vi "485测试事件结构.vi"() -> ()   [LabVIEW 2018]
doc: "本范例可设置指定端口的RS-485收发器控制模式，并实现串口读取、串口写入或串口读写操作。如果选择全部，VI将写入数据并读取数据，然后关闭开放给端口的VISA会话句柄。该VI将等待直到端口接收到指定的字节数或者接收到终止符。本范例仅适用于NI RS-485接口。\n\n范例演示了使用NI RS-485产品时可用的收发器控制模式。通过RS-485连接一个或多个设备时，用户可能需要减少连线数量。或者用户需要匹配部分设备提供的连线配置。根据连接串行设备所需的连线方式可确定NI RS-485收发器控制模式。\n\n与双线设备进行通信时，National Instruments建议使用双线自动控制模式。该模式可处理硬件中两线连接的发送器/接收器启用模式，因此可减少应用程序中执行该操作的软件开销。"
uses:
  <vilib>/Instr/_visa.llb/VISA Configure Serial Port (Instr).vi
panel:
  in  "时":dbl
  in  "分":dbl
  out "日期":string
  out "时间":string
  out "字符串":string
  in  "秒":dbl
  in  "停止 3":bool
  out "Serial Settings:Number of Bytes at Serial Port 5":u32
  in  "关闭全部继电器":bool=TRUE
  out "Serial Settings:Number of Bytes at Serial Port 4":u32
  in  "打开全部继电器":bool=TRUE
  out "Serial Settings:Number of Bytes at Serial Port 3":u32
  out "数字 2":u32
  out "数字":u32
  in  "停止":bool
  out "读取缓冲区":string
  in  "串口设置":T1={"baud rate"=9600, "data bits"=8, "parity"=enum."None", "stop bits"=10, "flow control"=0} {"flow control" items=["无"=0, "XON/XOFF"=1, "RTS/CTS"=2, "DTR/DSR"=4]; "stop bits" items=["1.0"=10, "1.5"=15, "2.0"=20]; "data bits" min=5 max=8 step=1; "baud rate" items=["75"=75, "110"=110, "134"=134, "150"=150, "300"=300, "600"=600, "1200"=1200, "1800"=1800, "2400"=2400, "4800"=4800, "7200"=7200, "9600"=9600, "14400"=14400, "19200"=19200, "28800"=28800, "38400"=38400, "56000"=56000, "57600"=57600, "115200"=115200, "128000"=128000, "230400"=230400]}
  in  "VISA RS 485资源":refnum<visa-resource-name>="COM1"
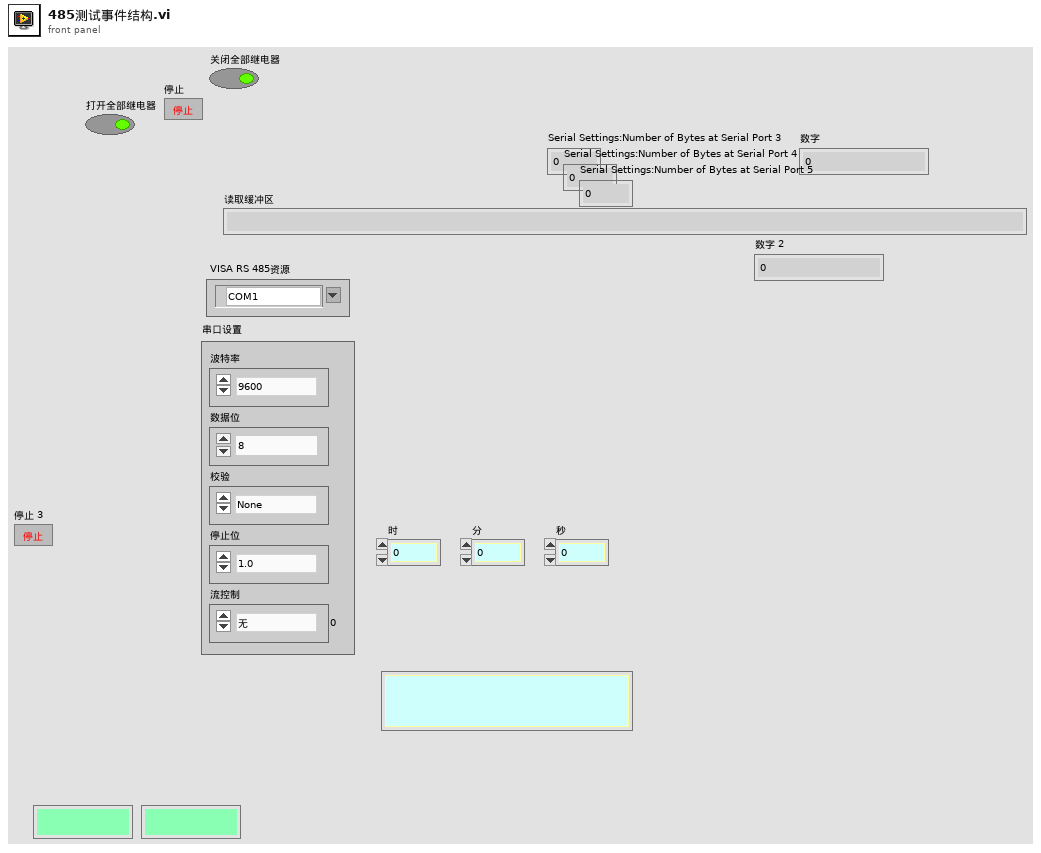
[diagram p1: front panel]
types:
  T1 = typedef "Serial - Settings.ctl" = cluster{"baud rate":u32, "data bits":u16, "parity":enum16{"None", "Odd", "Even", "Mark", "Space"}, "stop bits":u16, "flow control":u16}
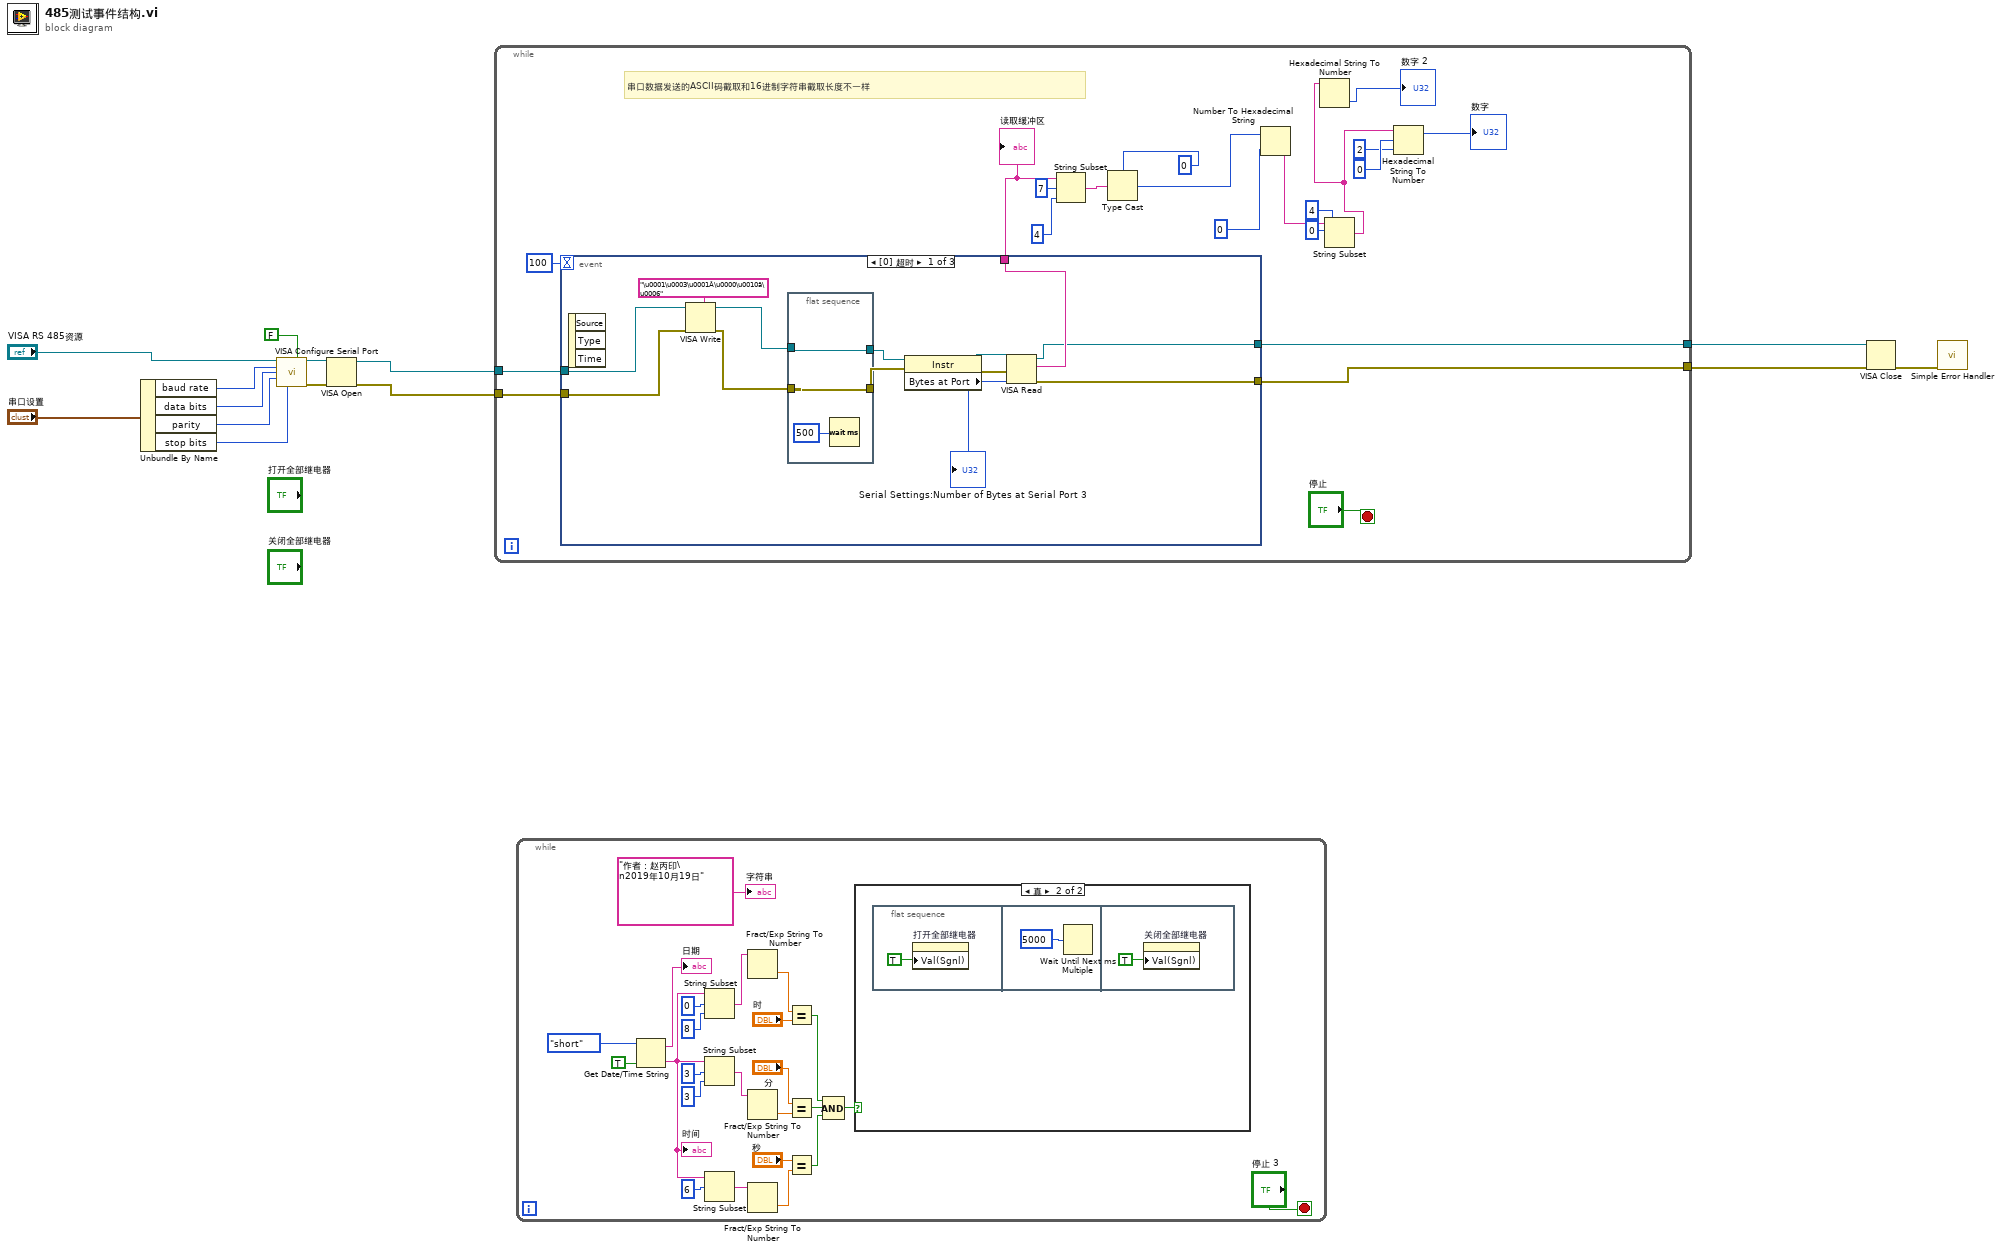
[diagram p0: block diagram]
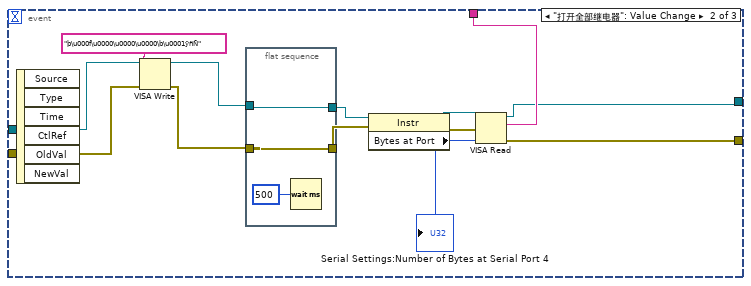
[diagram p3: hidden frame]
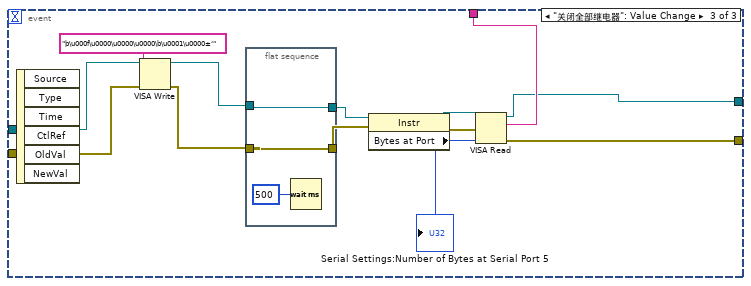
[diagram p4: hidden frame]
diagram:
  n1 = Unbundle By Name("串口设置") -> ("baud rate"=w12:u32, "data bits"=w11:u16, "parity"=w10:enum16{"None", "Odd", "Even", "Mark", "Space"}, "stop bits"=w9:u16)
  n2 = call-poly "VISA Configure Serial Port"("VISA resource name"="VISA RS 485资源", "Enable Termination\nChar (T)"=FALSE ("Enable Termination\nChar (T)"), "baud rate (9600)"=w12, "data bits (8)"=w11, "parity (0:none)"=w10, "stop bits (10: 1 bit)"=w9) -> ("VISA resource name out"=w3:refnum<visa-resource-name>, "error out"=w4:errorcluster)  [unwired: 3 in, 5 out]
  n3 = VISA Open(error in (no error)=w4, VISA resource name=w3) -> (VISA resource name=w1:refnum<visa-resource-name>, error out=w2:errorcluster)  [unwired: 3 in]
  n4 = while {
    tunnel: [w23] -> w6
    tunnel: [w22] -> w5
    tunnel: w2 -> [w18]
    tunnel: w1 -> [w17]
    stop <- "停止" stop-if-true
    # "串口数据发送的ASCII码截取和16进制字符串截取长度不一样"
    n5 = event shown="[0] 超时" {
      selector: _ -> [_ _ _]
      dyn-events: _ -> [_ _ _]
      timeout: 100 -> [_ _ _]
      tunnel: [w48 w64 w80] -> w34
      tunnel: [w47 w52 w68] -> w23
      tunnel: [w46 w53 w69] -> w22
      tunnel: w18 -> [w45 w63 w79]
      tunnel: w17 -> [w44 w62 w78]
      event Timeout {
        n6 = event-data() -> ()  [unwired: 1 in, 3 out]
        n7 = VISA Write(VISA resource name=w44, write buffer="\u0001\u0003\u0001Â\u0000\u0010ä\u0006" ("写入字符串 3"), error in (no error)=w45) -> (VISA resource name out=w39:refnum<visa-resource-name>, error out=w37:errorcluster)  [unwired: 1 out]
        n8 = flat-sequence {
          tunnel: w39 -> [w51]
          tunnel: [w51] -> w38
          tunnel: w37 -> [w50]
          tunnel: [w50] -> w36
          frame #0 {
            n9 = Wait (ms)(milliseconds to wait=u32 500 ("等待时间（毫秒）")) -> ()  [unwired: 1 out]
          }
        }
        n10 = property class="Instr"(reference=w38, error in=w36) -> (reference out=w41:refnum<visa-resource-name>, error out=w40:errorcluster, "Bytes at Port"=w42:u32)
        "Serial Settings:Number of Bytes at Serial Port 3" <- w42
        n11 = VISA Read(VISA resource name=w41, byte count=w42, error in (no error)=w40) -> (VISA resource name out=w46:refnum<visa-resource-name>, read buffer=w48:string, error out=w47:errorcluster)  [unwired: 1 out]
      }
      event "打开全部继电器": Value Change {
        n12 = event-data() -> ()  [unwired: 1 in, 6 out]
        n13 = VISA Write(VISA resource name=w62, write buffer="þ\u000f\u0000\u0000\u0000\b\u0001ÿñÑ" ("写入字符串 3"), error in (no error)=w63) -> (VISA resource name out=w57:refnum<visa-resource-name>, error out=w55:errorcluster)  [unwired: 1 out]
        n14 = flat-sequence {
          tunnel: w57 -> [w67]
          tunnel: [w67] -> w56
          tunnel: w55 -> [w66]
          tunnel: [w66] -> w54
          frame #0 {
            n15 = Wait (ms)(milliseconds to wait=u32 500 ("等待时间（毫秒）")) -> ()  [unwired: 1 out]
          }
        }
        n16 = property class="Instr"(reference=w56, error in=w54) -> (reference out=w59:refnum<visa-resource-name>, error out=w58:errorcluster, "Bytes at Port"=w60:u32)
        "Serial Settings:Number of Bytes at Serial Port 4" <- w60
        n17 = VISA Read(VISA resource name=w59, byte count=w60, error in (no error)=w58) -> (VISA resource name out=w53:refnum<visa-resource-name>, read buffer=w64:string, error out=w52:errorcluster)  [unwired: 1 out]
      }
      event "关闭全部继电器": Value Change {
        n18 = event-data() -> ()  [unwired: 1 in, 6 out]
        n19 = VISA Write(VISA resource name=w78, write buffer="þ\u000f\u0000\u0000\u0000\b\u0001\u0000±‘" ("写入字符串 3"), error in (no error)=w79) -> (VISA resource name out=w73:refnum<visa-resource-name>, error out=w71:errorcluster)  [unwired: 1 out]
        n20 = flat-sequence {
          tunnel: w73 -> [w83]
          tunnel: [w83] -> w72
          tunnel: w71 -> [w82]
          tunnel: [w82] -> w70
          frame #0 {
            n21 = Wait (ms)(milliseconds to wait=u32 500 ("等待时间（毫秒）")) -> ()  [unwired: 1 out]
          }
        }
        n22 = property class="Instr"(reference=w72, error in=w70) -> (reference out=w75:refnum<visa-resource-name>, error out=w74:errorcluster, "Bytes at Port"=w76:u32)
        "Serial Settings:Number of Bytes at Serial Port 5" <- w76
        n23 = VISA Read(VISA resource name=w75, byte count=w76, error in (no error)=w74) -> (VISA resource name out=w69:refnum<visa-resource-name>, read buffer=w80:string, error out=w68:errorcluster)  [unwired: 1 out]
      }
    }
    "读取缓冲区" <- w34
    n24 = String Subset(string=w34, offset (0)=7 ("偏移量(0)"), length (rest)=4 ("长度（剩余）")) -> (substring=w20:string)
    n25 = Type Cast(type=0, x=w20) -> (*(type *) &x=w30:i32)
    n26 = Number To Hexadecimal String(1:u32 0 ("宽度(-)"), 2:w30) -> (0:w19:string)
    n27 = String Subset(string=w19, offset (0)=0 ("偏移量(0)"), length (rest)=4 ("长度（剩余）")) -> (substring=w16:string)
    n28 = Hexadecimal String To Number(string=w16) -> (number=→"数字 2":u32)  [unwired: 2 in, 1 out]
    n29 = Hexadecimal String To Number(string=w16, offset=0 ("偏移量"), default (0uL)=u32 2 ("默认(0 U32)")) -> (number=→"数字":u32)  [unwired: 1 out]
  }
  n30 = while {
    stop <- "停止 3" stop-if-true
    n31 = Get Date/Time String(date format (0)=enum16{"short", "long", "abbreviated"}."short" ("日期格式(0)"), want seconds? (F)=TRUE) -> (date string=→"日期":string, time string=w90:string)  [unwired: 1 in]
    "时间" <- w90
    n32 = String Subset(string=w90, offset (0)=0, length (rest)=8) -> (substring=w103:string)
    n33 = String Subset(string=w90, offset (0)=3, length (rest)=3) -> (substring=w99:string)
    n34 = String Subset(string=w90, offset (0)=6) -> (substring=w98:string)  [unwired: 1 in]
    n35 = Fract/Exp String To Number(string=w103) -> (number=w97:dbl)  [unwired: 3 in, 1 out]
    n36 = Fract/Exp String To Number(string=w99) -> (number=w96:dbl)  [unwired: 3 in, 1 out]
    n37 = Fract/Exp String To Number(string=w98) -> (number=w86:dbl)  [unwired: 3 in, 1 out]
    n38 = Equal?(x=w97, y="时") -> (x = y?=w95:bool)
    n39 = Equal?(x="分", y=w96) -> (x = y?=w94:bool)
    n40 = Equal?(x="秒", y=w86) -> (x = y?=w87:bool)
    n41 = Compound Arithmetic op=AND(w95, w94, w87) -> (w84:bool)
    n42 = case shown="真" w84 {
      frame False {
      }
      frame True {
        n43 = flat-sequence {
          frame #0 {
            n44 = property on="打开全部继电器" class="Bool (严格)"("Val(Sgnl)"=TRUE ("值(信号)")) -> ()  [unwired: 2 in, 2 out]
          }
          frame #1 {
            n45 = Wait Until Next ms Multiple(millisecond multiple=u32 5000 ("毫秒倍数")) -> ()  [unwired: 1 out]
          }
          frame #2 {
            n46 = property on="关闭全部继电器" class="Bool (严格)"("Val(Sgnl)"=TRUE ("值(信号)")) -> ()  [unwired: 2 in, 2 out]
          }
        }
      }
    }
    "字符串" <- "作者：赵丙印\n2019年10月19日" ("字符串")
  }
  n47 = VISA Close(VISA resource name=w5, error in (no error)=w6) -> (error out=w7:errorcluster)
  n48 = call <vilib>:"Simple Error Handler.vi"("error in (no error)"=w7) -> ()  [unwired: 1 in, 8 out]
